vi "TCP_Server_loop.vi"(4 "error in (no error)":errorcluster, 6 "queue in":refnum<queue>, 7 "TCP Connection ID":refnum<k5>) -> (0 "error out":errorcluster, 3 "Shutdown?":bool)   [LabVIEW 2015]
uses:
  Systems/SystemUtil/Command.ctl
  Systems/Primary Filter/f1driveractions.ctl
  Systems/Secondary Filter/f2driveractions.ctl
  Systems/Coll_Focus/coll_actions.ctl
  Systems/Cam_Focus/CF_drivercontrol.ctl
  Systems/Grating_Translation/GTdriveractions.ctl
  Systems/Slit/slitactions.ctl
  Systems/Wavelength/wavelength_driver_actions.ctl
  Systems/Wavelength/wavelength_parameters.ctl
  Systems/Wavelength/movetypes.ctl
panel:
  out "Command History":string
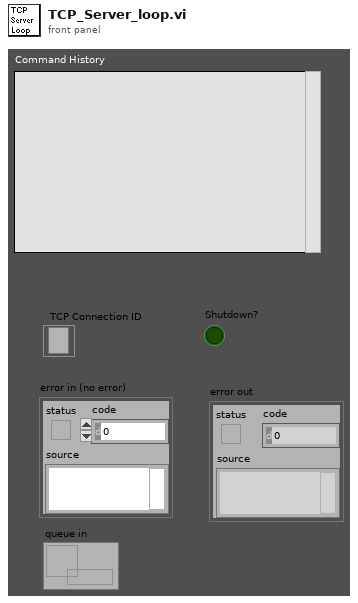
[diagram p1: front panel]
types:
  T1 = typedef "Command.ctl" = cluster{"Command":string, "Parameter":string}
  T2 = typedef "f1driveractions.ctl" = enum16{"Launch", "INIT_CTL", "Home", "Move", "Shutdown"}
  T3 = typedef "f2driveractions.ctl" = enum16{"Launch", "INIT_CTL", "Home", "Move", "Shutdown"}
  T4 = typedef "coll_actions.ctl" = enum16{"Launch", "Move", "Home", "Open Shutter", "Close Shutter", "Shutdown"}
  T5 = typedef "CF_drivercontrol.ctl" = enum16{"Launch", "Move", "Set Piezos", "Flexure On", "Flexure Off", "Home", "Shutdown"}
  T6 = typedef "GTdriveractions.ctl" = enum16{"Launch", "INIT_CTL", "Move", "Home", "Shutdown"}
  T7 = typedef "slitactions.ctl" = enum16{"Launch", "INIT_CTL", "Restart", "Show", "Hide", "Home", "Move", "Rotate Only", "Shutdown"}
  T8 = typedef "wavelength_parameters.ctl" = cluster{"Camera Angle":dbl, "Grating  Angle":dbl, "Move type":T9}
  T9 = typedef "movetypes.ctl" = u16
  T10 = typedef "wavelength_driver_actions.ctl" = enum16{"Launch", "Flexure On", "Flexure Off", "Move", "Home", "Shutdown"}
  T11 = typedef "ThreadStates.ctl" = enum16{"Waiting", "Scripting", "Uninitialized", "Error"}
  T12 = cluster{"GT Thread state":T11, "Slit Thread State":T11, "F1 Thread State":T11, "F2 Thread State":T11, "Coll Thread State":T11, "CF Thread State":T11, "Wavelength Thread State":T11}
  T13 = cluster{"Grating Name":string, "Slit Name":string, "Primary Filter Name":string, "Secondary Filter name":string, "Coll Position":i32, "Camera Focus":i32, "Camera Angle":dbl, "Grating Angle":dbl, "Coll Temp":dbl, "CF Temp\n":dbl, "Camera Target":dbl, "Grating Target":dbl, "WAVMODE":string, "Slit Hidden??":bool}
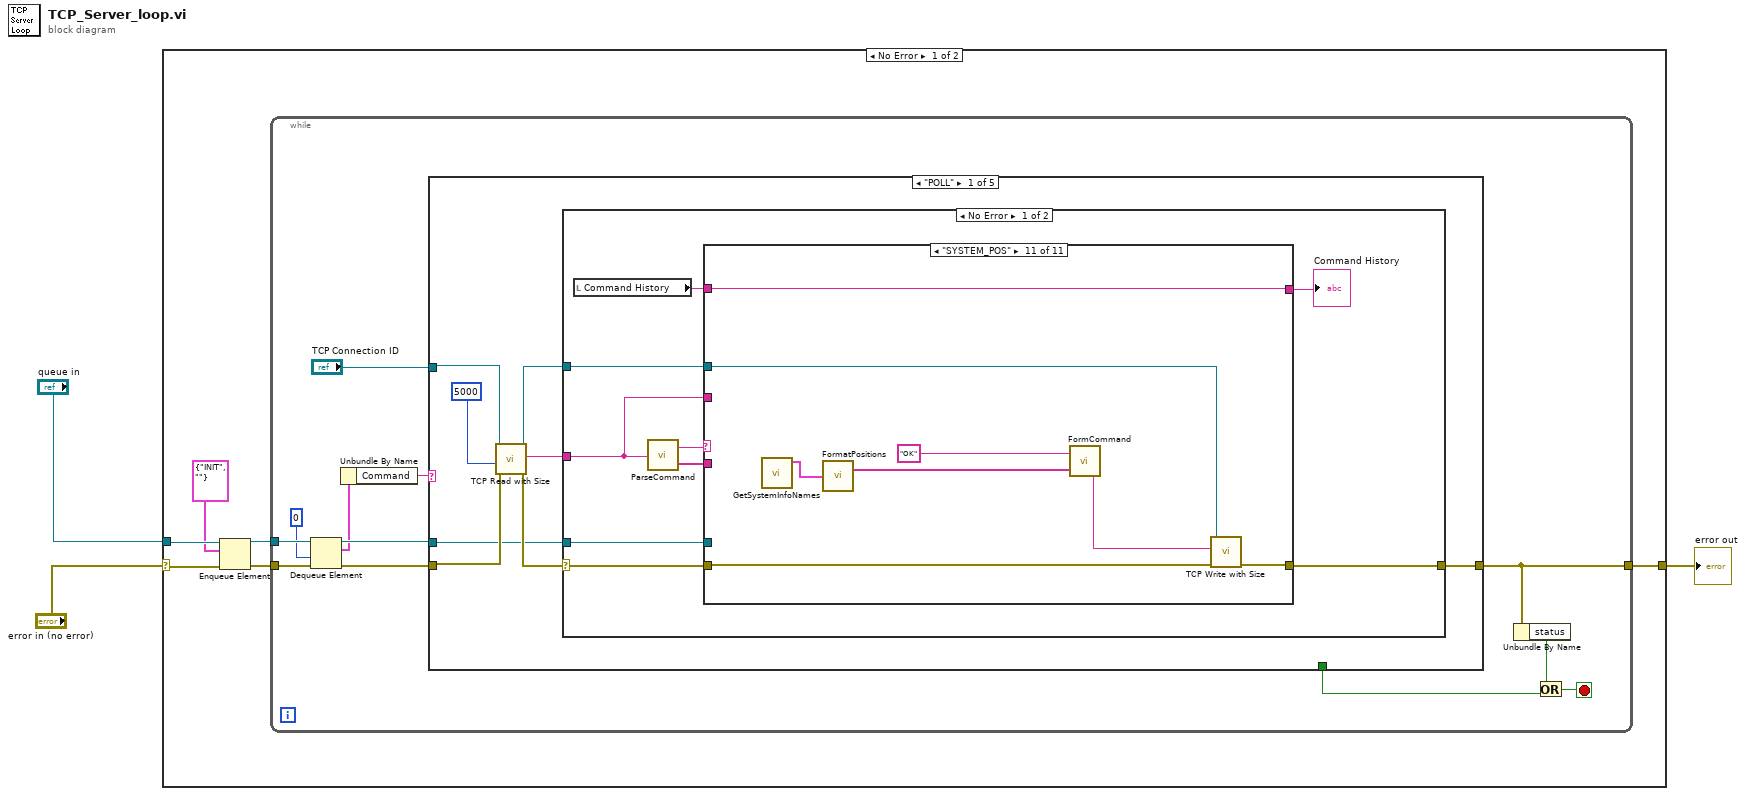
[diagram p0: block diagram]
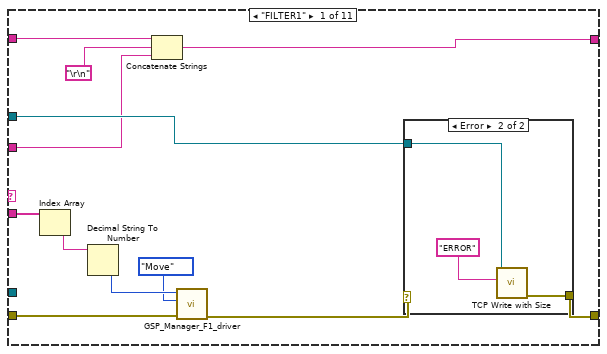
[diagram p2: hidden frame]
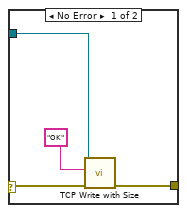
[diagram p3: hidden frame]
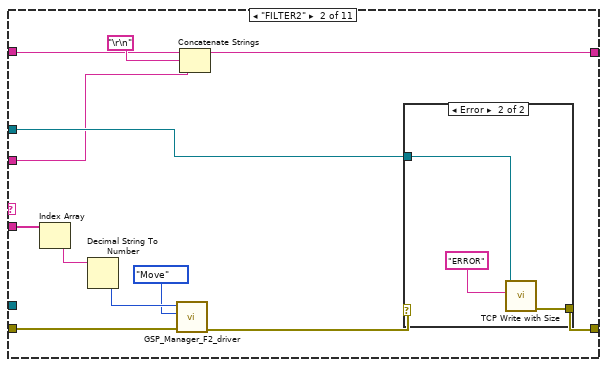
[diagram p4: hidden frame]
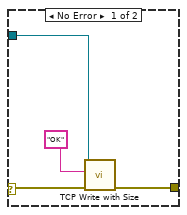
[diagram p5: hidden frame]
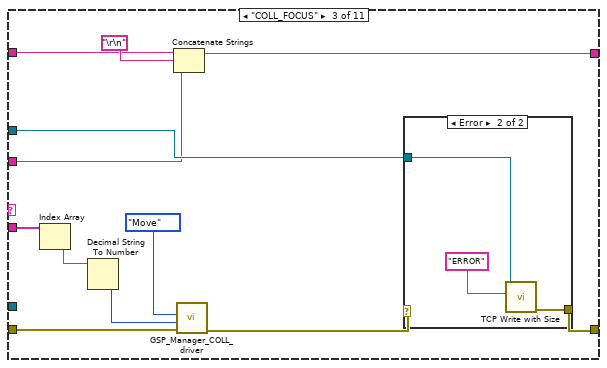
[diagram p6: hidden frame]
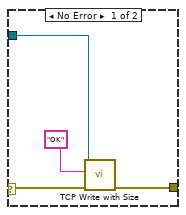
[diagram p7: hidden frame]
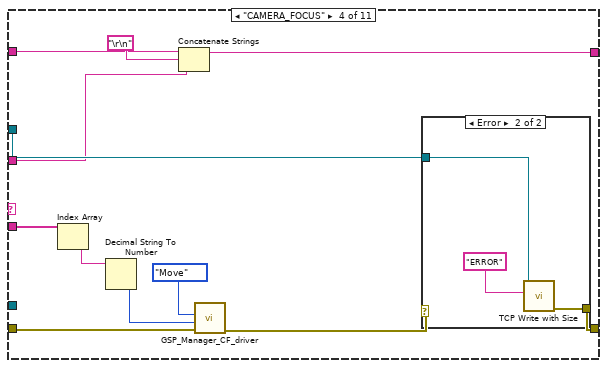
[diagram p8: hidden frame]
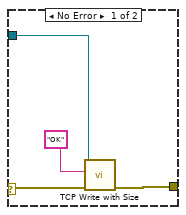
[diagram p9: hidden frame]
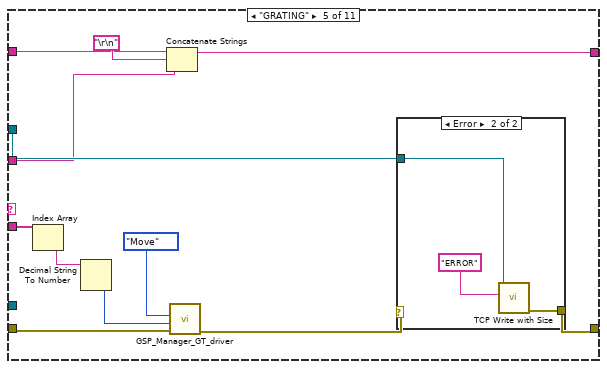
[diagram p10: hidden frame]
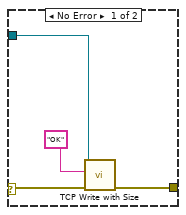
[diagram p11: hidden frame]
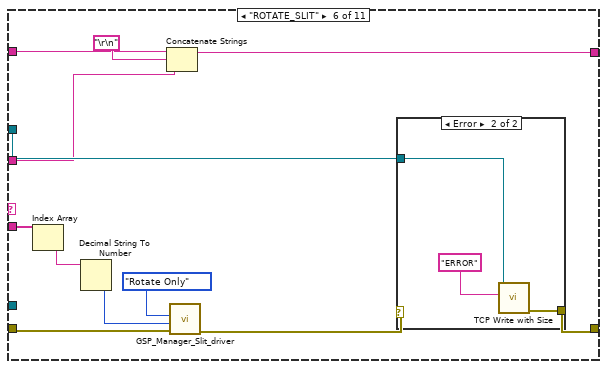
[diagram p12: hidden frame]
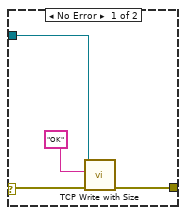
[diagram p13: hidden frame]
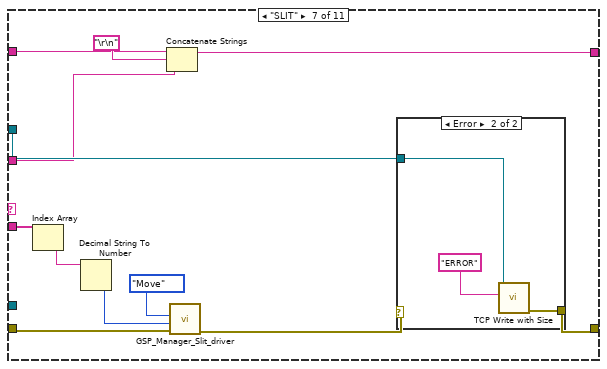
[diagram p14: hidden frame]
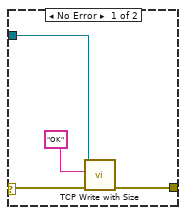
[diagram p15: hidden frame]
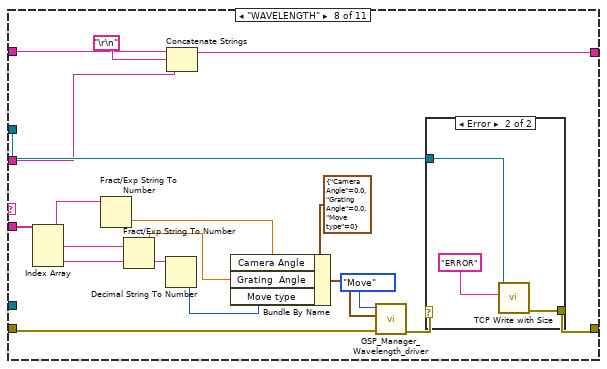
[diagram p16: hidden frame]
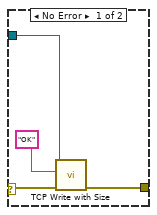
[diagram p17: hidden frame]
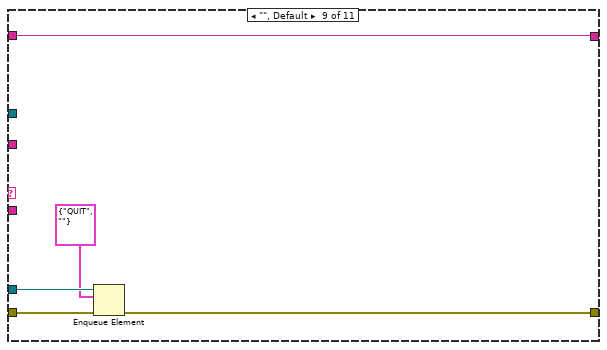
[diagram p18: hidden frame]
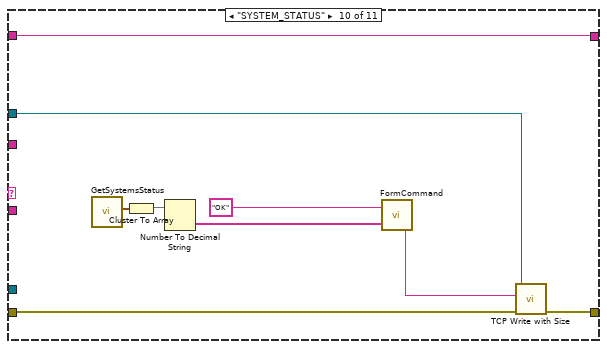
[diagram p19: hidden frame]
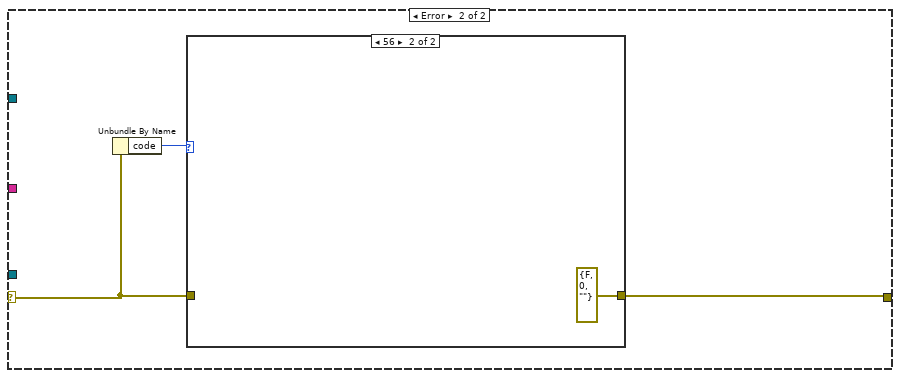
[diagram p20: hidden frame]
diagram:
  n1 = case shown="No Error" "error in (no error)" {
    selector: "error in (no error)" -> [w5 w245]
    tunnel: [w9 w245] -> w2
    tunnel: "queue in" -> [w6 _]
    frame No Error {
      n2 = Enqueue Element(queue=w6, element=T1 {"Command"="INIT", "Parameter"=""}, error in (no error)=w5) -> (queue out=w8:refnum<queue>, error out=w7:errorcluster)  [unwired: 1 in, 1 out]
      n3 = while {
        tunnel: w8 -> [w21]
        tunnel: [w16] -> w9
        tunnel: w7 -> [w13]
        stop <- w18 stop-if-true
        n4 = Dequeue Element(queue=w21, timeout in ms (-1)=0, error in (no error)=w13) -> (queue out=w19:refnum<queue>, element=w12:T1, error out=w20:errorcluster)  [unwired: 1 out]
        n5 = Unbundle By Name(w12) -> ("Command"=w11:string)
        n6 = case shown="\"POLL\"" w11 {
          tunnel: w19 -> [w22 w226 _ _ _]
          tunnel: w20 -> [w29 w227 w237 w241 w244]
          tunnel: "TCP Connection ID" -> [w28 _ w239 w240 _]
          tunnel: [w23 w224 w237 w241 w244] -> w16
          tunnel: [_ _ TRUE w242 _] -> w14
          frame "POLL" {
            n7 = call "TCP Read with Size.vi"("error in (no error)"=w29, "timeout ms (25000)"=5000, "connection ID"=w28) -> ("error out"=w24:errorcluster, "data out"=w26:string, "connection ID out"=w25:refnum<k5>)  [unwired: 6 in]
            n8 = case shown="No Error" w24 {
              selector: w24 -> [w34 w220]
              tunnel: w26 -> [w31 _]
              tunnel: w25 -> [w38 _]
              tunnel: [w33 w219] -> w23
              tunnel: w22 -> [w35 _]
              frame No Error {
                n9 = local read "Command History"() -> (w32:string)
                n10 = call "ParseCommand.vi"("Command string"=w31) -> ("Command"=w37:string, "Parameters"=w36:string[])
                n11 = case shown="\"SYSTEM_POS\"" w37 {
                  tunnel: w38 -> [w45 w65 w86 w104 w123 w142 w161 w187 _ w204 w215]
                  tunnel: w36 -> [w50 w69 w88 w101 w121 w140 w159 w185 _ _ _]
                  tunnel: w35 -> [_ _ _ _ _ _ _ _ w201 _ _]
                  tunnel: w34 -> [w48 w67 w82 w103 w122 w141 w160 w186 w200 w205 w216]
                  tunnel: [w44 w64 w85 w102 w119 w139 w158 w184 w198 w206 w217] -> w33
                  tunnel: w32 -> [w41 w60 w79 w98 w117 w137 w156 w182 w197 w202 w212]
                  tunnel: w31 -> [w40 w58 w77 w96 w115 w135 w154 w180 _ _ _]
                  tunnel: [w42 w59 w78 w97 w116 w136 w155 w181 w197 w202 w212] -> w30
                  frame "FILTER1" {
                    n12 = Index Array(array=w50) -> (element=w49:string)  [unwired: 1 in]
                    n13 = Decimal String To Number(string=w49) -> (number=w47:i32)  [unwired: 2 in, 1 out]
                    n14 = Concatenate Strings(w41, "\r\n", w40) -> (w42:string)
                    n15 = call "GSP_Manager_F1_driver.vi"("error in (no error)"=w48, "Action"=f1driveractions."Move", "Filter# (Move Only)"=w47) -> ("error out"=w43:errorcluster)  [unwired: 3 in, 1 out]
                    n16 = case shown="Error" w43 {
                      selector: w43 -> [w51 _]
                      tunnel: w45 -> [w53 w55]
                      tunnel: [w52 w56] -> w44
                      frame No Error {
                        n17 = call "TCP Write with Size.vi"("error in (no error)"=w51, "data in"="OK", "connection ID"=w53) -> ("error out"=w52:errorcluster)  [unwired: 6 in, 2 out]
                      }
                      frame Error {
                        n18 = call "TCP Write with Size.vi"("data in"="ERROR", "connection ID"=w55) -> ("error out"=w56:errorcluster)  [unwired: 7 in, 2 out]
                      }
                    }
                  }
                  frame "FILTER2" {
                    n19 = Index Array(array=w69) -> (element=w68:string)  [unwired: 1 in]
                    n20 = Decimal String To Number(string=w68) -> (number=w66:i32)  [unwired: 2 in, 1 out]
                    n21 = call "GSP_Manager_F2_driver.vi"("error in (no error)"=w67, "Action"=f2driveractions."Move", "Filter# (Move Only)"=w66) -> ("error out"=w63:errorcluster)  [unwired: 3 in, 1 out]
                    n22 = Concatenate Strings(w60, "\r\n", w58) -> (w59:string)
                    n23 = case shown="Error" w63 {
                      selector: w63 -> [w70 _]
                      tunnel: w65 -> [w72 w75]
                      tunnel: [w71 w74] -> w64
                      frame No Error {
                        n24 = call "TCP Write with Size.vi"("error in (no error)"=w70, "data in"="OK", "connection ID"=w72) -> ("error out"=w71:errorcluster)  [unwired: 6 in, 2 out]
                      }
                      frame Error {
                        n25 = call "TCP Write with Size.vi"("data in"="ERROR", "connection ID"=w75) -> ("error out"=w74:errorcluster)  [unwired: 7 in, 2 out]
                      }
                    }
                  }
                  frame "COLL_FOCUS" {
                    n26 = Index Array(array=w88) -> (element=w87:string)  [unwired: 1 in]
                    n27 = Decimal String To Number(string=w87) -> (number=w84:i32)  [unwired: 2 in, 1 out]
                    n28 = Concatenate Strings(w79, "\r\n", w77) -> (w78:string)
                    n29 = call "GSP_Manager_COLL_driver.vi"("error in (no error)"=w82, "Target (Move Only)"=w84, "Action"=coll_actions."Move") -> ("error out"=w81:errorcluster)  [unwired: 3 in, 1 out]
                    n30 = case shown="Error" w81 {
                      selector: w81 -> [w89 _]
                      tunnel: w86 -> [w91 w94]
                      tunnel: [w90 w93] -> w85
                      frame No Error {
                        n31 = call "TCP Write with Size.vi"("error in (no error)"=w89, "data in"="OK", "connection ID"=w91) -> ("error out"=w90:errorcluster)  [unwired: 6 in, 2 out]
                      }
                      frame Error {
                        n32 = call "TCP Write with Size.vi"("data in"="ERROR", "connection ID"=w94) -> ("error out"=w93:errorcluster)  [unwired: 7 in, 2 out]
                      }
                    }
                  }
                  frame "CAMERA_FOCUS" {
                    n33 = Index Array(array=w101) -> (element=w107:string)  [unwired: 1 in]
                    n34 = Decimal String To Number(string=w107) -> (number=w106:i32)  [unwired: 2 in, 1 out]
                    n35 = Concatenate Strings(w98, "\r\n", w96) -> (w97:string)
                    n36 = call "GSP_Manager_CF_driver.vi"("error in (no error)"=w103, "Target (Move Only)"=w106, "Action"=CF_drivercontrol."Move") -> ("error out"=w105:errorcluster)  [unwired: 4 in, 1 out]
                    n37 = case shown="Error" w105 {
                      selector: w105 -> [w108 _]
                      tunnel: w104 -> [w110 w113]
                      tunnel: [w109 w112] -> w102
                      frame No Error {
                        n38 = call "TCP Write with Size.vi"("error in (no error)"=w108, "data in"="OK", "connection ID"=w110) -> ("error out"=w109:errorcluster)  [unwired: 6 in, 2 out]
                      }
                      frame Error {
                        n39 = call "TCP Write with Size.vi"("data in"="ERROR", "connection ID"=w113) -> ("error out"=w112:errorcluster)  [unwired: 7 in, 2 out]
                      }
                    }
                  }
                  frame "GRATING" {
                    n40 = Index Array(array=w121) -> (element=w126:string)  [unwired: 1 in]
                    n41 = Decimal String To Number(string=w126) -> (number=w125:i32)  [unwired: 2 in, 1 out]
                    n42 = Concatenate Strings(w117, "\r\n", w115) -> (w116:string)
                    n43 = call "GSP_Manager_GT_driver.vi"("error in (no error)"=w122, "Grating # (Move Only)"=w125, "Action"=GTdriveractions."Move") -> ("error out"=w124:errorcluster)  [unwired: 3 in, 1 out]
                    n44 = case shown="Error" w124 {
                      selector: w124 -> [w127 _]
                      tunnel: w123 -> [w129 w132]
                      tunnel: [w128 w131] -> w119
                      frame No Error {
                        n45 = call "TCP Write with Size.vi"("error in (no error)"=w127, "data in"="OK", "connection ID"=w129) -> ("error out"=w128:errorcluster)  [unwired: 6 in, 2 out]
                      }
                      frame Error {
                        n46 = call "TCP Write with Size.vi"("data in"="ERROR", "connection ID"=w132) -> ("error out"=w131:errorcluster)  [unwired: 7 in, 2 out]
                      }
                    }
                  }
                  frame "ROTATE_SLIT" {
                    n47 = Index Array(array=w140) -> (element=w145:string)  [unwired: 1 in]
                    n48 = Decimal String To Number(string=w145) -> (number=w144:i32)  [unwired: 2 in, 1 out]
                    n49 = Concatenate Strings(w137, "\r\n", w135) -> (w136:string)
                    n50 = call "GSP_Manager_Slit_driver.vi"("error in (no error)"=w141, "Slit # (Move/Rotate Only)"=w144, "Action"=slitactions."Rotate Only") -> ("error out"=w143:errorcluster)  [unwired: 3 in, 1 out]
                    n51 = case shown="Error" w143 {
                      selector: w143 -> [w146 _]
                      tunnel: w142 -> [w148 w151]
                      tunnel: [w147 w150] -> w139
                      frame No Error {
                        n52 = call "TCP Write with Size.vi"("error in (no error)"=w146, "data in"="OK", "connection ID"=w148) -> ("error out"=w147:errorcluster)  [unwired: 6 in, 2 out]
                      }
                      frame Error {
                        n53 = call "TCP Write with Size.vi"("data in"="ERROR", "connection ID"=w151) -> ("error out"=w150:errorcluster)  [unwired: 7 in, 2 out]
                      }
                    }
                  }
                  frame "SLIT" {
                    n54 = Index Array(array=w159) -> (element=w164:string)  [unwired: 1 in]
                    n55 = Decimal String To Number(string=w164) -> (number=w163:i32)  [unwired: 2 in, 1 out]
                    n56 = Concatenate Strings(w156, "\r\n", w154) -> (w155:string)
                    n57 = call "GSP_Manager_Slit_driver.vi"("error in (no error)"=w160, "Slit # (Move/Rotate Only)"=w163, "Action"=slitactions."Move") -> ("error out"=w162:errorcluster)  [unwired: 3 in, 1 out]
                    n58 = case shown="Error" w162 {
                      selector: w162 -> [w165 _]
                      tunnel: w161 -> [w167 w170]
                      tunnel: [w166 w169] -> w158
                      frame No Error {
                        n59 = call "TCP Write with Size.vi"("error in (no error)"=w165, "data in"="OK", "connection ID"=w167) -> ("error out"=w166:errorcluster)  [unwired: 6 in, 2 out]
                      }
                      frame Error {
                        n60 = call "TCP Write with Size.vi"("data in"="ERROR", "connection ID"=w170) -> ("error out"=w169:errorcluster)  [unwired: 7 in, 2 out]
                      }
                    }
                  }
                  frame "WAVELENGTH" {
                    n61 = Index Array(array=w185) -> (element #1=w189:string, element #2=w178:string, element #3=w177:string)  [unwired: 3 in]
                    n62 = Fract/Exp String To Number(string=w189) -> (number=w174:dbl)  [unwired: 3 in, 1 out]
                    n63 = Fract/Exp String To Number(string=w178) -> (number=w173:dbl)  [unwired: 3 in, 1 out]
                    n64 = Decimal String To Number(string=w177) -> (number=w172:i32)  [unwired: 2 in, 1 out]
                    n65 = Concatenate Strings(w182, "\r\n", w180) -> (w181:string)
                    n66 = Bundle By Name(cluster=T8 {"Camera Angle"=0.0, "Grating  Angle"=0.0, "Move type"=0} ("Target (Move Only)"), "Camera Angle"=w174, "Grating  Angle"=w173, "Move type"=w172) -> (w175:T8)
                    n67 = call "GSP_Manager_Wavelength_driver.vi"("error in (no error)"=w186, "Target (Move Only)"=w175, "Action"=wavelength_driver_actions."Move") -> ("error out"=w188:errorcluster)  [unwired: 3 in, 1 out]
                    n68 = case shown="Error" w188 {
                      selector: w188 -> [w190 _]
                      tunnel: w187 -> [w192 w195]
                      tunnel: [w191 w194] -> w184
                      frame No Error {
                        n69 = call "TCP Write with Size.vi"("error in (no error)"=w190, "data in"="OK", "connection ID"=w192) -> ("error out"=w191:errorcluster)  [unwired: 6 in, 2 out]
                      }
                      frame Error {
                        n70 = call "TCP Write with Size.vi"("data in"="ERROR", "connection ID"=w195) -> ("error out"=w194:errorcluster)  [unwired: 7 in, 2 out]
                      }
                    }
                  }
                  frame "", Default {
                    n71 = Enqueue Element(queue=w201, element=T1 {"Command"="QUIT", "Parameter"=""}, error in (no error)=w200) -> (error out=w198:errorcluster)  [unwired: 1 in, 2 out]
                  }
                  frame "SYSTEM_STATUS" {
                    n72 = call "GetSystemsStatus.vi"() -> ("Thread States"=w210:T12)  [unwired: 4 in, 3 out]
                    n73 = Cluster To Array(cluster=w210) -> (array=w209:T11[])
                    n74 = Number To Decimal String(number=w209) -> (decimal integer string=w208:string[])  [unwired: 1 in]
                    n75 = call "FormCommand.vi"("Parameters"=w208, "Command"="OK") -> ("Command string"=w203:string)
                    n76 = call "TCP Write with Size.vi"("error in (no error)"=w205, "data in"=w203, "connection ID"=w204) -> ("error out"=w206:errorcluster)  [unwired: 6 in, 2 out]
                  }
                  frame "SYSTEM_POS" {
                    n77 = call "GetSystemInfoNames.vi"() -> ("Pos Info"=w211:T13)  [unwired: 11 in]
                    n78 = call "FormatPositions.vi"("Pos Info"=w211) -> ("Pos strings"=w214:string[])
                    n79 = call "FormCommand.vi"("Parameters"=w214, "Command"="OK") -> ("Command string"=w213:string)
                    n80 = call "TCP Write with Size.vi"("error in (no error)"=w216, "data in"=w213, "connection ID"=w215) -> ("error out"=w217:errorcluster)  [unwired: 6 in, 2 out]
                  }
                }
                "Command History" <- w30
              }
              frame Error {
                n81 = Unbundle By Name(w220) -> ("code"=w221:i32)
                n82 = case shown="56" w221 {
                  tunnel: w220 -> [w222 _]
                  tunnel: [w222 errorcluster {"status"=FALSE, "code"=0, "source"=""} ("error IO")] -> w219
                  frame 0, Default {
                  }
                  frame 56 {
                  }
                }
              }
            }
          }
          frame "", Default {
            n83 = event shown="[1] Panel Close?" {
              selector: _ -> [_ _]
              dyn-events: _ -> [_ _]
              timeout: 0 -> [_ _]
              tunnel: w227 -> [w230 w234]
              tunnel: w226 -> [w231 w235]
              tunnel: [w228 w233] -> w224
              event Timeout {
                n84 = event-data() -> ()  [unwired: 1 in, 2 out]
                n85 = Enqueue Element(queue=w231, element=T1 {"Command"="POLL", "Parameter"=""}, error in (no error)=w230) -> (error out=w228:errorcluster)  [unwired: 1 in, 2 out]
              }
              event Panel Close? {
                n86 = event-data() -> ()  [unwired: 1 in, 4 out]
                n87 = Enqueue Element(queue=w235, element=T1 {"Command"="QUIT", "Parameter"=""}, error in (no error)=w234) -> (error out=w233:errorcluster)  [unwired: 1 in, 2 out]
                n88 = event-data("Discard?"=TRUE) -> ()  [unwired: 1 in, 1 out]
              }
            }
          }
          frame "QUIT" {
            n89 = TCP Close Connection(connection ID=w239) -> ()  [unwired: 2 in, 2 out]
          }
          frame "SHUTDOWN" {
            w242 = TRUE
            n90 = TCP Close Connection(connection ID=w240) -> ()  [unwired: 2 in, 2 out]
            "Shutdown?" <- w242
          }
          frame "INIT" {
            n91 = local write "Command History"("") -> ()
          }
        }
        n92 = Unbundle By Name(w16) -> ("status"=w15:bool)
        n93 = Or(x=w15, y=w14) -> (x .or. y?=w18:bool)
      }
    }
    frame Error {
    }
  }
  "error out" <- w2
